vi "Initialize HW Interface.vi"(0 "Hardware Interface in":refnum<class "Hardware Interface.lvclass">, 5 "HW Interface Names":T3, 7 "Buttons Names":cluster{"name":string[], "type":T2[]}, 9 "Interpolation Coefficients":T1, 11 "error in (no error)":errorcluster) -> (4 "Hardware Interface out":refnum<class "Hardware Interface.lvclass">, 15 "error out":errorcluster)   [LabVIEW 2013, in "Hardware Interface.lvclass"]
uses:
  Hardware Interface.lvclass
  ButtonType.ctl
  <vilib>/Analysis/Matrix/Datatypes/RealMatrix.ctl
  Hardware Interface.lvclass/Hardware Interface.ctl
  <vilib>/Analysis/Matrix/NI_Matrix.lvlib
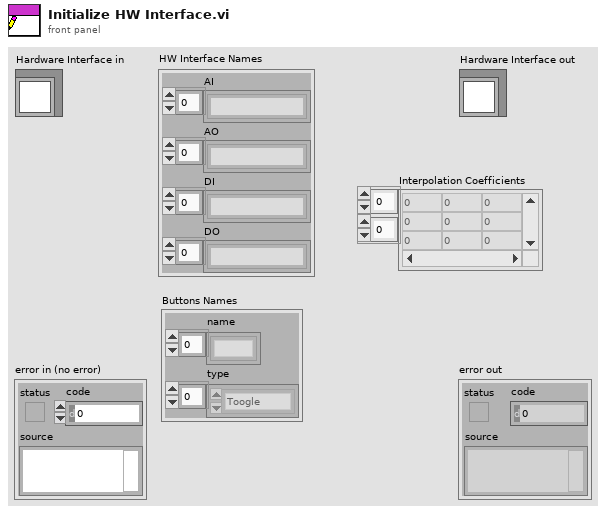
[diagram p1: front panel]
types:
  T1 = typedef "NI_Matrix.lvlib/RealMatrix.ctl" = dbl[][]
  T2 = typedef "ButtonType.ctl" = enum16{"Toogle", "Switch"}
  T3 = cluster{"AI":string[], "AO":string[], "DI":string[], "DO":string[]}
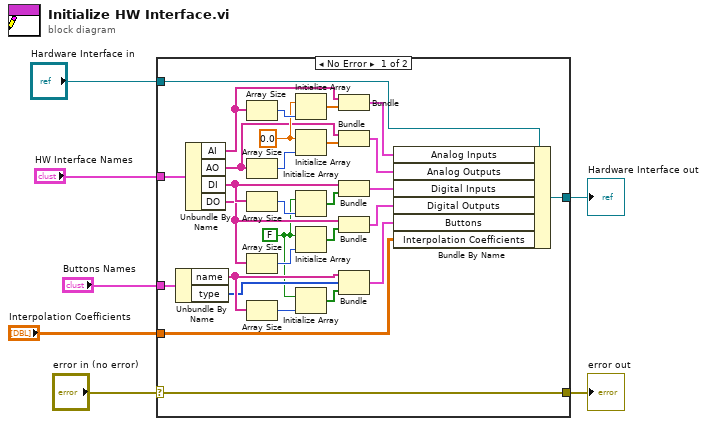
[diagram p0: block diagram]
diagram:
  n1 = case shown="No Error" "error in (no error)" {
    selector: "error in (no error)" -> [w36 w37]
    tunnel: [w36 w37] -> w6
    tunnel: [w34 w38] -> w4
    tunnel: "Hardware Interface in" -> [w35 w38]
    tunnel: "Interpolation Coefficients" -> [w33 _]
    tunnel: "HW Interface Names" -> [w32 _]
    tunnel: "Buttons Names" -> [w14 _]
    frame No Error {
      w10 = FALSE
      w23 = 0.0 ("element")
      n2 = Unbundle By Name(w14) -> ("name"=w13:string[], "type"=w12:T2[])
      n3 = Unbundle By Name(w32) -> ("AI"=w30:string[], "AO"=w22:string[], "DI"=w20:string[], "DO"=w16:string[])
      n4 = Array Size(array=w30) -> (size(s)=w31:i32)
      n5 = Array Size(array=w22) -> (size(s)=w24:i32)
      n6 = Array Size(array=w20) -> (size(s)=w19:i32)
      n7 = Array Size(array=w16) -> (size(s)=w15:i32)
      n8 = Array Size(array=w13) -> (size(s)=w9:i32)
      n9 = Initialize Array(w23, w31) -> (w29:dbl[])
      n10 = Initialize Array(w23, w24) -> (w21:dbl[])
      n11 = Initialize Array(w10, w19) -> (w18:bool[])
      n12 = Initialize Array(w10, w15) -> (w17:bool[])
      n13 = Initialize Array(w10, w9) -> (w8:bool[])
      n14 = Bundle("AI"=w30, w29) -> (w28:cluster{"AI":string[], dbl[]})  [unwired: 1 in]
      n15 = Bundle("AO"=w22, w21) -> (w27:cluster{"AO":string[], dbl[]})  [unwired: 1 in]
      n16 = Bundle("DI"=w20, w18) -> (w26:cluster{"DI":string[], bool[]})  [unwired: 1 in]
      n17 = Bundle("DO"=w16, w17) -> (w25:cluster{"DO":string[], bool[]})  [unwired: 1 in]
      n18 = Bundle("name"=w13, "type"=w12, w8) -> (w11:cluster{"name":string[], "type":T2[], bool[]})  [unwired: 1 in]
      n19 = Bundle By Name(cluster=w35, "Analog Inputs"=w28, "Analog Outputs"=w27, "Digital Inputs"=w26, "Digital Outputs"=w25, "Buttons"=w11, "Interpolation Coefficients"=w33) -> (w34:refnum<class "Hardware Interface.lvclass">)
    }
    frame Error {
    }
  }
  "error out" <- w6
  "Hardware Interface out" <- w4
